vi "Create 16B RT FIFO.vi"(7 "size (10)":u32=10, 8 "error in (no error)":errorcluster) -> (0 "error out":errorcluster, 3 "RT FIFO":T1)   [LabVIEW 2017, in "Data Sharing Framework Engine.lvlib" / "Engine Interface.lvclass"]
uses:
  Engine Interface.lvclass
  16B RT FIFO Reference.ctl
  16B Data.ctl
  16B Payload.ctl
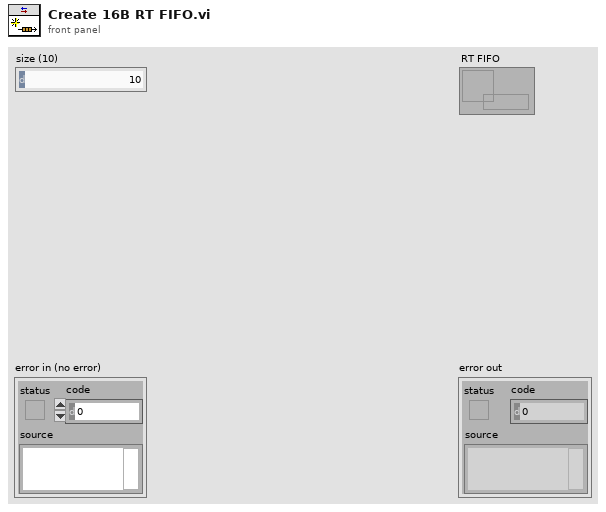
[diagram p1: front panel]
types:
  T1 = typedef "Data Sharing Framework Engine.lvlib/Engine Interface.lvclass/16B RT FIFO Reference.ctl" = refnum<k33>
  T2 = cluster{"read mode":enum16{"polling", "blocking"}, "write mode":enum16{"polling", "blocking"}}
  T3 = typedef "Data Sharing Framework Engine.lvlib/Engine Interface.lvclass/16B Data.ctl" = cluster{"Command":u8, "Payload":T4}
  T4 = typedef "Data Sharing Framework Engine.lvlib/Engine Interface.lvclass/16B Payload.ctl" = cluster{"arg1":u64, "arg2":u64}
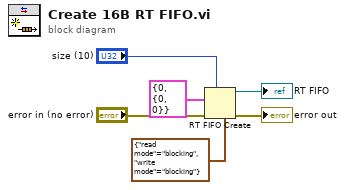
[diagram p0: block diagram]
diagram:
  n1 = RT FIFO Create(1:T3 {"Command"=0, "Payload"={"arg1"=0, "arg2"=0}} ("Cluster"), 3:"error in (no error)", 4:"size (10)", 7:T2 {"read mode"=enum."blocking", "write mode"=enum."blocking"} ("r/w modes (polling,polling)")) -> (8:→"RT FIFO":refnum<k33>, 11:→"error out":errorcluster)  [unwired: 4 in, 1 out]
